vi "Open API Tester.vi"(8 "error in":errorcluster, 11 "DQMH Library Ref":refnum<vi>) -> (0 "error out":errorcluster)   [LabVIEW 2019, in "Panther Dashboard.lvlib"]
doc: "This VI checks the Main.vi State of the selected DQMH Module"
uses:
  Panther Dashboard.lvlib
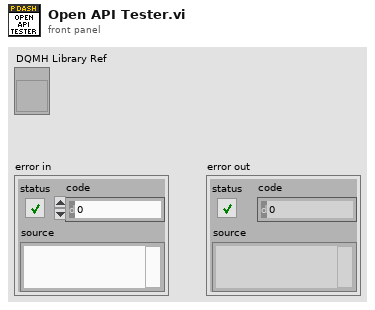
[diagram p1: front panel]
types:
  T1 = enum32{"Bad", "Idle", "Run top level", "Running"}
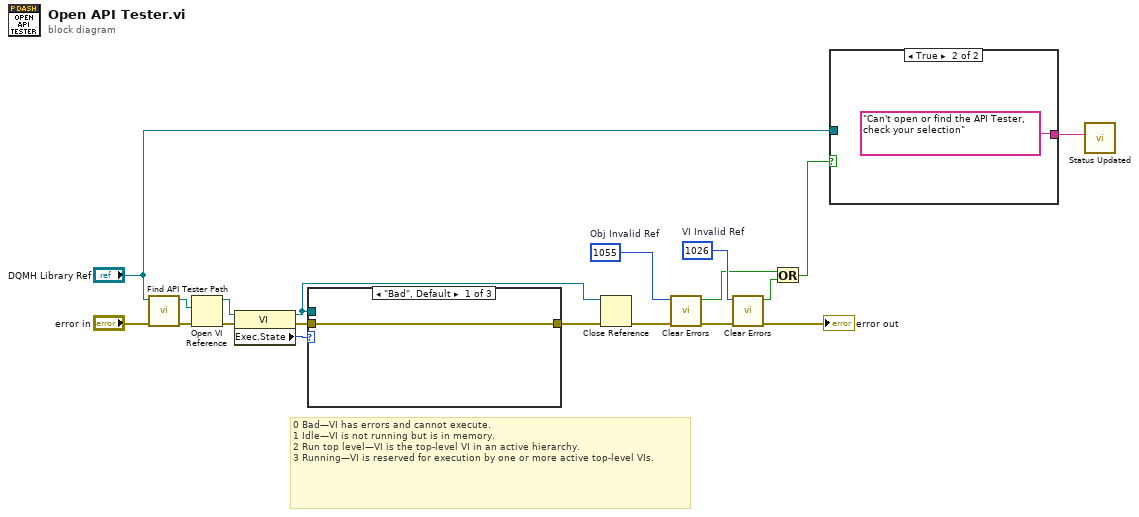
[diagram p0: block diagram]
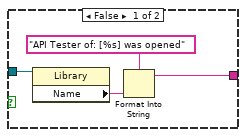
[diagram p2: hidden frame]
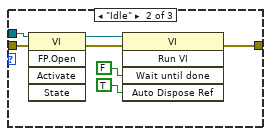
[diagram p3: hidden frame]
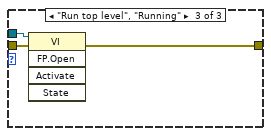
[diagram p4: hidden frame]
diagram:
  w7 = 1055  # Obj Invalid Ref
  w6 = 1026  # VI Invalid Ref
  # "0\tBad—VI has errors and cannot execute.\n1\tIdle—VI is not running but is in memory.\n2\tRun top level—VI is the top-level VI in an active hierarchy.\n3\tRunning—VI is reserved for execution by one or more active top-level VIs."
  n1 = call "Find API Tester Path.vi"("error in"="error in", "DQMH Library Ref"="DQMH Library Ref") -> ("error out"=w17:errorcluster, "API Tester Path"=w11:path)  [unwired: 8 in]
  n2 = Open VI Reference(vi path=w11, error in (no error)=w17) -> (vi reference=w10:refnum<vi>, error out=w19:errorcluster)  [unwired: 4 in]
  n3 = property class="VI"(reference=w10, error in=w19) -> (reference out=w8:refnum<vi>, error out=w16:errorcluster, "Exec.State"=w9:T1)
  n4 = case shown="\"Bad\", Default" w9 {
    tunnel: w8 -> [_ w21 w28]
    tunnel: w16 -> [w20 w26 w29]
    tunnel: [w20 w25 w30] -> w15
    frame "Bad", Default {
    }
    frame "Idle" {
      n5 = invoke class="VI" method="FP.Open"(reference=w21, error in=w26) -> (reference out=w24:refnum<vi>, error out=w27:errorcluster)  [unwired: 3 in, 3 out]
      n6 = invoke class="VI" method="Run VI"(reference=w24, error in=w27, "Wait until done"=FALSE ("Wait Until Done"), "Auto Dispose Ref"=TRUE ("Auto Dispose Reference")) -> (error out=w25:errorcluster)  [unwired: 1 in, 4 out]
    }
    frame "Run top level", "Running" {
      n7 = invoke class="VI" method="FP.Open"(reference=w28, error in=w29) -> (error out=w30:errorcluster)  [unwired: 3 in, 4 out]
    }
  }
  n8 = Close Reference(reference=w8, error in (no error)=w15) -> (error out=w14:errorcluster)
  n9 = call <vilib>:"Clear Errors.vi"("error in (no error)"=w14, "specific error code to clear (0: all)"=w7) -> ("error out"=w13:errorcluster, "specific error cleared?"=w5:bool)  [unwired: 4 in]
  n10 = call <vilib>:"Clear Errors.vi"("error in (no error)"=w13, "specific error code to clear (0: all)"=w6) -> ("error out"=→"error out":errorcluster, "specific error cleared?"=w4:bool)  [unwired: 4 in]
  n11 = Or(x=w5, y=w4) -> (x .or. y?=w3:bool)
  n12 = case shown="True" w3 {
    tunnel: "DQMH Library Ref" -> [w32 _]
    tunnel: [w31 "Can't open or find the API Tester, check your selection"] -> w1
    frame False {
      n13 = property on="Property Node" class="Library"(reference=w32) -> ("Name"=w33:string)  [unwired: 1 in, 2 out]
      n14 = Format Into String(format string="API Tester of: [%s] was opened" ("Status"), w33) -> (resulting string=w31:string)  [unwired: 2 in, 1 out]
    }
    frame True {
    }
  }
  n15 = call "Status Updated.vi"("Status"=w1) -> ()  [unwired: 10 in, 1 out]
